vi "Halvorsen_MEMP_SVI.vi"(0 "Шаг h, с":ext, 1 "n":i32[](array[numeric]), 2 "k":i32, 3 "Parameter_Vector":ext[](array[numeric]), 5 "Время, с":ext, 7 "Initial Conditions":ext[](array[numeric]), 9 "Hmin":ext, 12 "Hmax":ext, 13 "tolerance":ext) -> (4 "Solution":ext[][](array[numeric]))   [LabVIEW 2016]
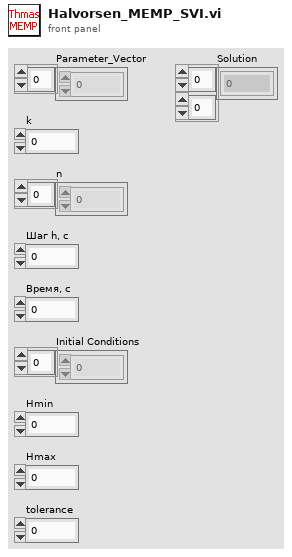
[diagram p1: front panel]
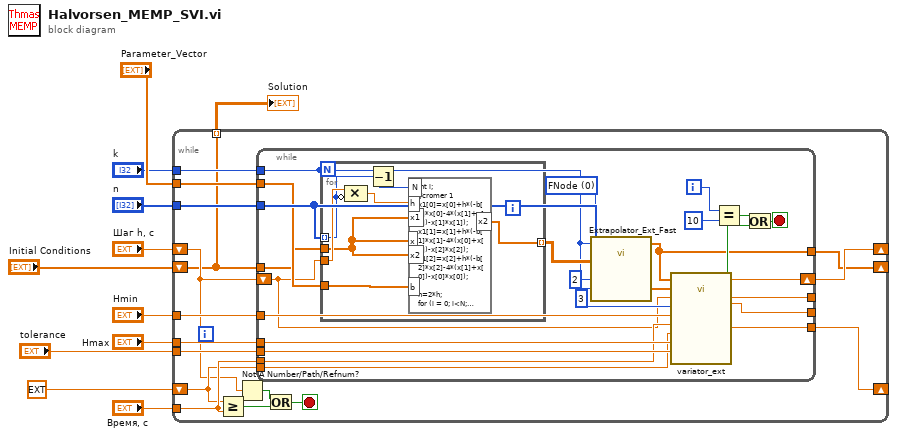
[diagram p0: block diagram]
diagram:
  n1 = while {
    shift-right: [w21] -> _
    shift-left: "Initial Conditions" -> [w12]
    tunnel: "n" -> [w27]
    tunnel: "k" -> [w26]
    shift-right: [w22] -> _
    shift-left: "Шаг h, с" -> [w14]
    shift-right: [w18] -> _
    shift-left: ext 0.0 -> [w19]
    tunnel: "Время, с" -> [w20]
    tunnel: "tolerance" -> [w23]
    tunnel: "Hmin" -> [w25]
    tunnel: "Hmax" -> [w24]
    tunnel: [w12] -> w9 mode=indexing
    tunnel: "Parameter_Vector" -> [w17]
    stop <- w16 stop-if-true
    n2 = Greater Or Equal?(x=w19, y=w20) -> (x >= y?=w15:bool)
    n3 = Not A Number/Path/Refnum?(number/path/refnum=w14) -> (NaN/Path/Refnum?=w13:bool)
    n4 = while {
      tunnel: w25 -> [w48]
      tunnel: w24 -> [w49]
      tunnel: w23 -> [w47]
      tunnel: w26 -> [w32]
      tunnel: w27 -> [w33]
      tunnel: w12 -> [w30]
      shift-right: [w42] -> w22
      shift-left: w14 -> [w29]
      tunnel: [w29] -> _
      tunnel: [w41] -> _
      tunnel: [w40] -> w21
      tunnel: w20 -> [w39]
      tunnel: w19 -> [w38]
      tunnel: [w36] -> w18
      tunnel: w17 -> [w31]
      i -> [w37]
      stop <- w43 stop-if-true
      w28 = u16 0 items=["FNode", "MathScript", "ECD8 Arrays", "ECD8 Fnode", "ECD8 FnodeDiv"] ("Ext.Type")
      n5 = for {
        N: w32 -> [_]
        tunnel: w33 -> [w57] mode=indexing
        tunnel: w29 -> [w58]
        tunnel: w30 -> [w53]
        tunnel: [w56] -> w34 mode=indexing
        tunnel: w31 -> [w52]
        n6 = Compound Arithmetic op=MULTIPLY(w58, invert w57) -> (w54:ext)
        n7 = Decrement(x=w57) -> (x-1=w55:i32)
        n8 = formula code="int i;\n//cromer 1\nx1[0]=x[0]+h*(-b[0]*x[0]-4*(x[1]+x[2])-x[1]*x[1]);\nx1[1]=x[1]+h*(-b[1]*x[1]-4*(x[0]+x[2])-x[2]*x[2]);\nx1[2]=x[2]+h*(-b[2]*x[2]-4*(x[1]+x[0])-x[0]*x[0]);\n\nh=2*h;\nfor (i = 0; i<N; i++)\n{\n//EEuler\nx2[0]=x[0]+h*(-b[0]*x1[0]-4*(x1[1]+x1[2])-x1[1]*x1[1]);\nx2[1]=x[1]+h*(-b[1]*x1[1]-4*(x1[0]+x1[2])-x1[2]*x1[2]);\nx2[2]=x[2]+h*(-b[2]*x1[2]-4*(x1[1]+x1[0])-x1[0]*x1[0]);\n\nx[0]=x1[0];\nx[1]=x1[1];\nx[2]=x1[2];\nx1[0]=x2[0];\nx1[1]=x2[1];\nx1[2]=x2[2];\n};\n\nh=h*0.5;\nx2[0]=(x[0]+x1[0]+h*(-b[0]*x1[0]-4*(x1[1]+x1[2])-x1[1]*x1[1]))/2;\nx2[1]=(x[1]+x1[1]+h*(-b[1]*x1[1]-4*(x1[0]+x1[2])-x1[2]*x1[2]))/2;\nx2[2]=(x[2]+x1[2]+h*(-b[2]*x1[2]-4*(x1[1]+x1[0])-x1[0]*x1[0]))/2;"("x"=w53, "x1"=w53, "h"=w54, "x2"=w53, "N"=w55, "b"=w52) -> ("x2"=w56:ext[])
      }
      n9 = call "Extrapolator_Ext_Fast.vi"("Порядок экстраполятора"=2 ("Ext. Order"), "Dimension"=3 ("input variable"), "Ext.Type"=w28, "Х - нач. условия"=w34, "n"=w33, "k"=w32) -> ("TPrev"=w50:ext[], "Tout"=w40:ext[])  [unwired: 4 in]
      n10 = call "variator_ext.vi"("Tout"=w40, "tolerance"=w47, "Hmax"=w49, "TPrev"=w50, "Шаг h, с"=w29, "Current time"=w38, "k"=w32, "Hmin"=w48, "tmax"=w39) -> ("Hnew"=w42:ext, "error estimation"=w41:ext, "New time"=w36:ext, "stop"=w44:bool)  [unwired: 3 in]
      n11 = Equal?(x=w37, y=10) -> (x = y?=w45:bool)
      n12 = Or(x=w45, y=w44) -> (x .or. y?=w43:bool)
    }
    n13 = Or(x=w13, y=w15) -> (x .or. y?=w16:bool)
  }
  "Solution" <- w9
